vi "EnqueueError.vi"(8 "Error Array In":errorcluster[](array[cluster]), 11 "Queue in":refnum<queue>) -> (0 "Error Array Out":errorcluster[](array[cluster]), 3 "Queue out":refnum<queue>)   [LabVIEW 2018, in "Visualization.lvlib" / "VisualizeBase.lvclass"]
doc: "This VI enqueues any error(s) that occurs."
uses:
  VisualizeBase/VisualizeBase_class/VisualizeBase.lvclass
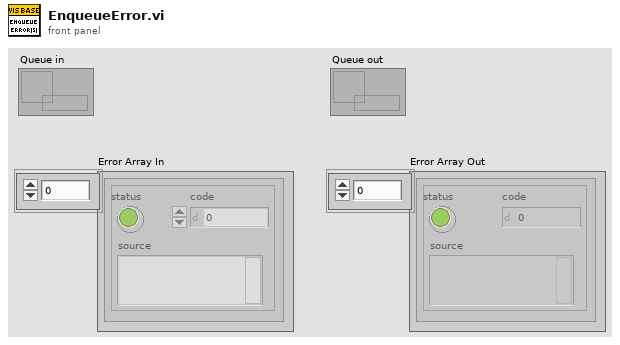
[diagram p1: front panel]
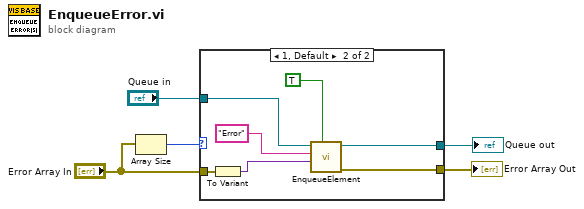
[diagram p0: block diagram]
diagram:
  n1 = Array Size(array="Error Array In") -> (size(s)=w5:i32)
  n2 = case shown="1, Default" w5 {
    tunnel: [w7 w13] -> w3
    tunnel: "Error Array In" -> [w7 w14]
    tunnel: "Queue in" -> [w6 w9]
    tunnel: [w6 w8] -> w1
    frame 0 {
    }
    frame 1, Default {
      n3 = To Variant(anything=w14) -> (Variant=w12:variant)
      n4 = call "EnqueueElement.vi"("Priority? (F)"=TRUE, "Data"=w12, "Message"="Error", "queue in"=w9) -> ("Error Array Out"=w13:errorcluster[], "queue out"=w8:refnum<queue>)  [unwired: 6 in]
    }
  }
  "Error Array Out" <- w3
  "Queue out" <- w1
